vi "Read User Apps.vi"(8 "error in (no error)":errorcluster) -> (0 "error out":errorcluster, 3 "User App Paths":path[](array[path]))   [LabVIEW 2020, in "PicoG-App.lvlib" / "App.lvclass"]
uses:
  App.lvclass
  PicoG-App.lvlib
  <vilib>/Utility/config.llb/NI_LVConfig.lvlib
  <vilib>/Utility/config.llb/Read Key (I32).vi
  <vilib>/Utility/config.llb/Read Key (Path).vi
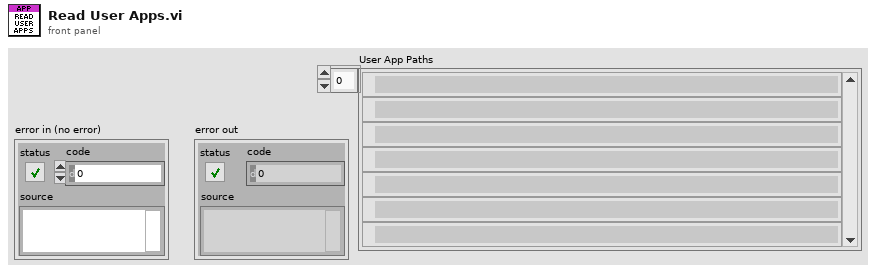
[diagram p1: front panel]
types:
  T1 = typedef "PicoG-App.lvlib/Paths.ctl" = cluster{"User picoG":path, "System picoG":path, "User Config":path, "System Config":path}
  T2 = typedef "NI_LVConfig.lvlib/Config Data RefNum.ctl" = refnum<k1>
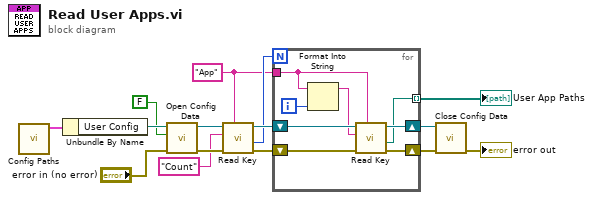
[diagram p0: block diagram]
diagram:
  w6 = "App" ("section")
  n1 = call "Config Paths.vi"() -> ("Paths"=w15:T1)  [unwired: 8 in, 3 out]
  n2 = Unbundle By Name(w15) -> ("User Config"=w14:path)
  n3 = call <vilib>:"Open Config Data.vi"("error in (no error)"="error in (no error)", "create file if necessary (T)"=FALSE, "configuration file path"=w14) -> ("error out"=w11:errorcluster, "refnum"=w12:T2)  [unwired: 6 in, 1 out]
  n4 = call-poly <vilib>:"Read Key.vi"("section"=w6, "error in (no error)"=w11, "key"="Count", "refnum"=w12) -> ("error out"=w8:errorcluster, "value"=w7:i32, "refnum out"=w9:T2)  [unwired: 4 in, 1 out]
  n5 = for {
    N: w7 -> [_]
    shift-right: [w18] -> w4
    shift-left: w9 -> [w22]
    shift-right: [w17] -> w3
    shift-left: w8 -> [w21]
    tunnel: w6 -> [w19]
    tunnel: [w16] -> w5 mode=indexing
    i -> [w23]
    n6 = Format Into String(initial string=w19, w23) -> (resulting string=w20:string)  [unwired: 2 in, 1 out]
    n7 = call-poly <vilib>:"Read Key.vi"("section"=w19, "error in (no error)"=w21, "key"=w20, "refnum"=w22) -> ("error out"=w17:errorcluster, "value"=w16:path, "refnum out"=w18:T2)  [unwired: 4 in, 1 out]
  }
  "User App Paths" <- w5
  n8 = call <vilib>:"Close Config Data.vi"("error in (no error)"=w3, "refnum"=w4) -> ("error out"=→"error out":errorcluster)  [unwired: 8 in, 1 out]
